vi "FPGA Reclosing Logic.vi"(0 "start reclaim timing? (T)":bool=TRUE, 1 "reclosing settings":T2={"number of reclosing attempts"=3, "dead times [ms]"=[200, 11000, 10000, 0, 0, 0, 0], "close pulse duration [ms]"=100, "reclaim time [ms]"=3000, "enable synchronism check? (F)"=FALSE, "enable lockout reset? (F)"=FALSE, "lockout reset time [ms]"=5000} {"number of reclosing attempts" items=["1"=1, "2"=2, "3"=3, "4"=4, "5"=5, "6"=6, "7"=7]}, 2 "reset? (F)":bool, 5 "trigger shot? (F)":bool, 7 "force to lockout state? (F)":bool, 9 "block close pulse? (F)":bool, 11 "synchronism check passed? (F)":bool) -> (4 "reclosing status":T1, 6 "shot count":u8, 8 "dead state?":bool, 10 "close pulse?":bool)   [LabVIEW 2013, in "NI_EP_Protection_FPGA.lvlib"]
doc: "Controls the automatic reclosing and lockout of a circuit breaker based on the reclosing settings that you specify. This VI also displays the reclosing status."
uses:
  <vilib>/addons/Electrical Power/Protection/NI_EP_Protection_FPGA.lvlib
  <vilib>/addons/Electrical Power/Protection/Reclosing Logic/subVIs/fpga_Recloser Logic Setting.ctl
  <vilib>/addons/Electrical Power/Protection/Reclosing Logic/subVIs/fpga_Recloser Sequence Status.ctl
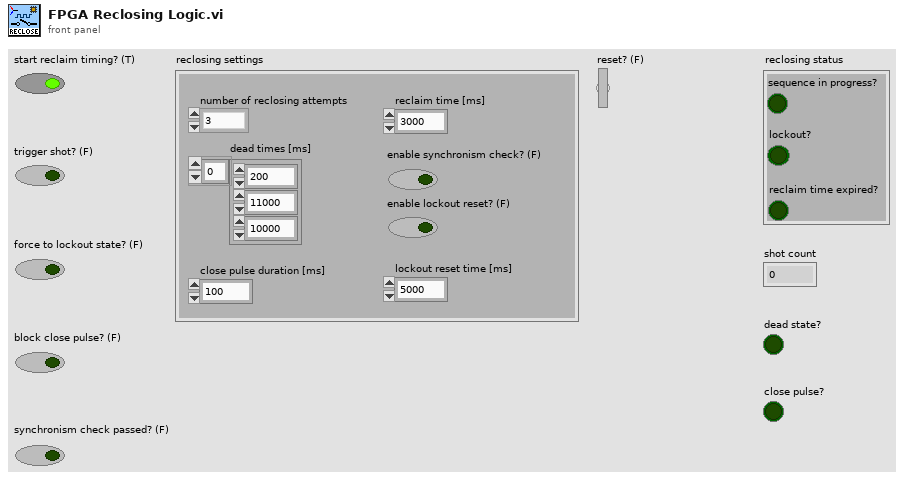
[diagram p1: front panel]
types:
  T1 = typedef "NI_EP_Protection_FPGA.lvlib/fpga_Recloser Sequence Status.ctl" = cluster{"sequence in progress?":bool, "lockout?":bool, "reclaim time expired?":bool}
  T2 = typedef "NI_EP_Protection_FPGA.lvlib/fpga_Recloser Logic Setting.ctl" = cluster{"number of reclosing attempts":u8, "dead times [ms]":u32[], "close pulse duration [ms]":u32, "reclaim time [ms]":u32, "enable synchronism check? (F)":bool, "enable lockout reset? (F)":bool, "lockout reset time [ms]":u32}
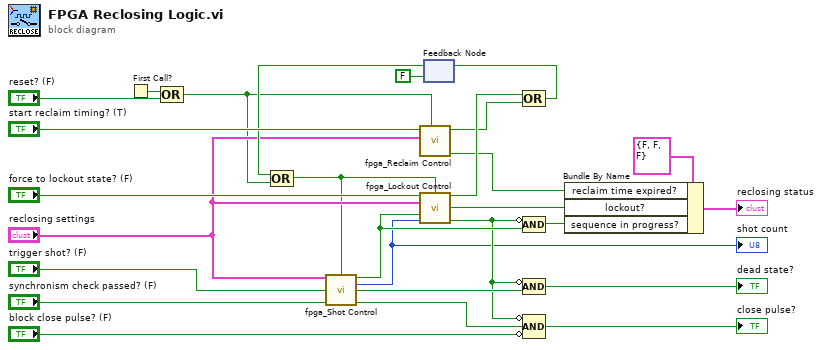
[diagram p0: block diagram]
diagram:
  n1 = First Call?() -> (First Call?: T/F=w5:bool)
  n2 = Compound Arithmetic op=OR(w5, "reset? (F)") -> (w3:bool)
  n3 = call <vilib>:"fpga_Reclaim Control.vi"("reset element? (F)"=w3, "reclosing setting"="reclosing settings", "break status? (T)"="start reclaim timing? (T)") -> ("reclaim time expired?"=w1:bool, "reclaim time expired pulse?"=w11:bool)  [unwired: 7 in]
  n4 = feedback #1(FALSE) -> (w10:bool)
  n5 = Compound Arithmetic op=OR(w10, w3) -> (w2:bool)
  n6 = call <vilib>:"fpga_Shot Control.vi"("reclosing setting"="reclosing settings", "reset to ready state? (F)"=w2, "shot trip? (F)"="trigger shot? (F)", "synchronism check pass? (F)"="synchronism check passed? (F)") -> ("sequence timer active?"=w16:bool, "shot count out"=w8:u8, "dead state?"=w14:bool, "close pulse signal"=w18:bool)  [unwired: 8 in]
  "shot count" <- w8
  n7 = call <vilib>:"fpga_Lockout Control.vi"("force to lockout state? (F)"="force to lockout state? (F)", "release from lockout? (F)"=w2, "reclosing setting"="reclosing settings", "sequence timer active? (F)"=w16, "shot count"=w8) -> ("released from lockout?"=w20:bool, "lockout?"=w17:bool, "block output during lockout?"=w12:bool)  [unwired: 8 in]
  n8 = Compound Arithmetic op=OR(w20, w11) -> (w24:bool)
  n9 = feedback-in #1(w24) -> ()
  n10 = Compound Arithmetic op=AND(invert w12, w16) -> (w15:bool)
  n11 = Compound Arithmetic op=AND(invert w12, w14) -> (→"dead state?":bool)
  n12 = Compound Arithmetic op=AND(invert w12, w18, invert "block close pulse? (F)") -> (→"close pulse?":bool)
  n13 = Bundle By Name(cluster=T1 {"sequence in progress?"=FALSE, "lockout?"=FALSE, "reclaim time expired?"=FALSE} ("reclosing status"), "reclaim time expired?"=w1, "lockout?"=w17, "sequence in progress?"=w15) -> (→"reclosing status":T1)
